vi "Create.vi"(8 "error in (no error)":errorcluster, 11 "This VI":refnum<vi>) -> (0 "error out":errorcluster, 3 "Budgetizer out":refnum<class "Budgetizer.lvclass">)   [LabVIEW 2018, in "Budgetizer.lvclass"]
uses:
  Budgetizer.lvclass
  Budgetizer.lvclass/Budgetizer.ctl
  database/Database.lvclass
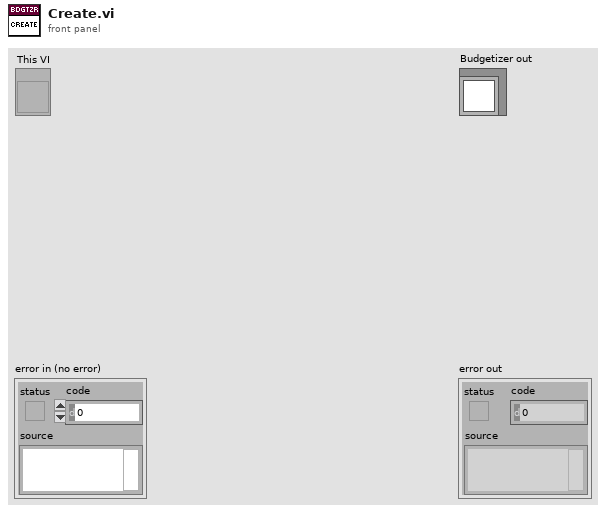
[diagram p1: front panel]
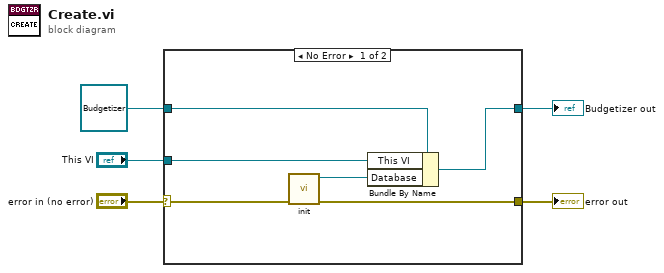
[diagram p0: block diagram]
diagram:
  n1 = case shown="No Error" "error in (no error)" {
    selector: "error in (no error)" -> [w7 w13]
    tunnel: [w8 w13] -> w4
    tunnel: [w10 w12] -> w2
    tunnel: refnum<class "Budgetizer.lvclass"> refnum ("Budgetizer in") -> [w11 w12]
    tunnel: "This VI" -> [w6 _]
    frame No Error {
      n2 = call "init.vi"("error in (no error)"=w7) -> ("error out"=w8:errorcluster, "Database.lvclass"=w9:refnum<class "Database.lvclass">)  [unwired: 9 in]
      n3 = Bundle By Name(cluster=w11, "This VI"=w6, "Database"=w9) -> (w10:refnum<class "Budgetizer.lvclass">)
    }
    frame Error {
    }
  }
  "error out" <- w4
  "Budgetizer out" <- w2
